vi "Create_Analogue_Time_Array.vi"(0 "Sampling Rate (Hz)":dbl, 1 "Sync Delay (s)":dbl, 2 "No of Samples":i32, 3 "Index":i32, 4 "Total No of Chs":i32) -> (5 "Times":dbl[](array[numeric]))   [LabVIEW 2017]
uses:
  Globals/Meas_global.vi
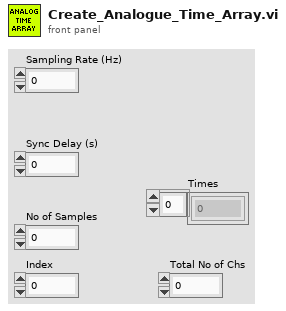
[diagram p1: front panel]
types:
  T1 = typedef "Trigger_Mode.ctl" = enum16{"Free Running", "Start on Trigger", "Trigger Every Block", "Trigger Every Sample"}
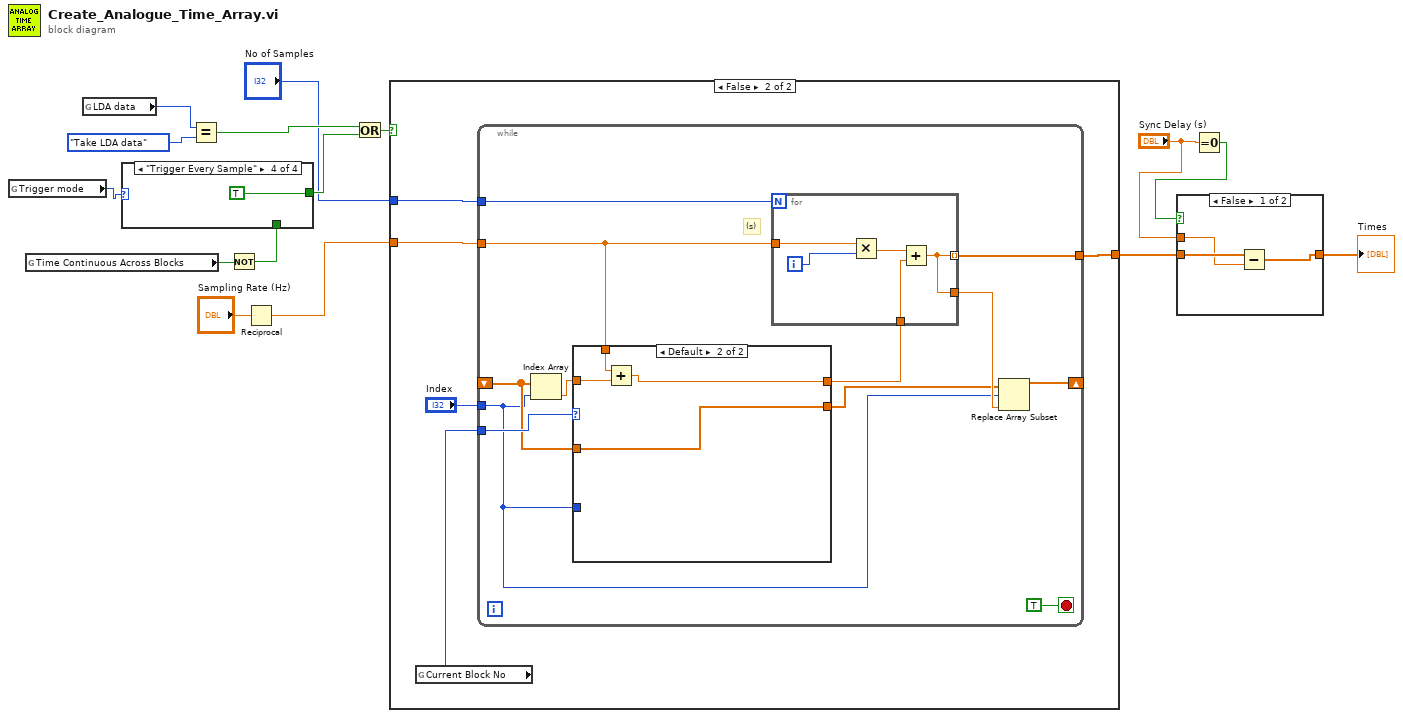
[diagram p0: block diagram]
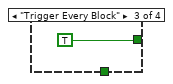
[diagram p5: hidden frame]
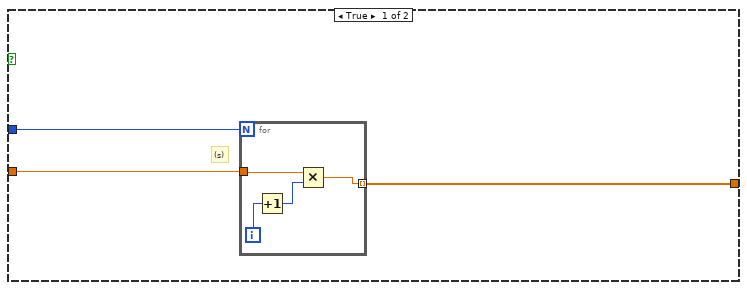
[diagram p6: hidden frame]
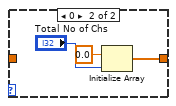
[diagram p8: hidden frame]
diagram:
  n1 = global read "Meas_global.vi" "Trigger mode"() -> (w14:T1)
  n2 = global read "Meas_global.vi" "Time Continuous Across Blocks"() -> (w9:bool)
  n3 = global read "Meas_global.vi" "LDA data"() -> (w6:enum16{"No LDA data", "Take LDA data"})
  n4 = Equal?(x=w6, y=enum16{"No LDA data", "Take LDA data"}."Take LDA data" ("LDA data")) -> (x = y?=w11:bool)
  n5 = Not(x=w9) -> (.not. x?=w8:bool)
  n6 = case shown="\"Trigger Every Sample\"" w14 {
    tunnel: [w16 w17 TRUE TRUE] -> w10
    tunnel: w8 -> [w16 w17 _ _]
    frame "Free Running" {
    }
    frame "Start on Trigger" {
    }
    frame "Trigger Every Block" {
    }
    frame "Trigger Every Sample" {
    }
  }
  n7 = Reciprocal(x="Sampling Rate (Hz)") -> (1/x=w15:dbl)
  n8 = Or(x=w11, y=w10) -> (x .or. y?=w12:bool)
  n9 = case shown="False" w12 {
    tunnel: [w22 w31] -> w2
    tunnel: "No of Samples" -> [w21 w30]
    tunnel: w15 -> [w20 w29]
    frame True {
      # "(s)"
      n10 = for {
        N: w21 -> [_]
        tunnel: w20 -> [w25]
        tunnel: [w24] -> w22 mode=indexing
        i -> [w26]
        n11 = Increment(x=w26) -> (x+1=w23:i32)
        n12 = Multiply(x=w25, y=w23) -> (x*y=w24:dbl)
      }
    }
    frame False {
      n13 = global read "Meas_global.vi" "Current Block No"() -> (w28:i32)
      n14 = while {
        tunnel: [w43] -> w31
        tunnel: w30 -> [w39]
        tunnel: w29 -> [w41]
        shift-right: [w38] -> _
        shift-left: _ -> [w33]
        tunnel: w28 -> [w40]
        tunnel: "Index" -> [w32]
        stop <- TRUE stop-if-true
        # "(s)"
        n15 = Index Array(array=w33, index=w32) -> (element=w36:dbl)
        n16 = case shown="Default" w40 {
          tunnel: [w47 w53] -> w37
          tunnel: w36 -> [_ w55]
          tunnel: w41 -> [w47 w54]
          tunnel: [w46 w52] -> w34
          tunnel: w33 -> [w44 w52]
          tunnel: w32 -> [w45 _]
          frame 1 {
            n17 = case shown="Default" w45 {
              tunnel: [w48 w49] -> w46
              tunnel: w44 -> [w48 _]
              frame Default {
              }
              frame 0 {
                n18 = Initialize Array(0.0 ("element"), "Total No of Chs") -> (w49:dbl[])
              }
            }
          }
          frame Default {
            n19 = Add(x=w54, y=w55) -> (x+y=w53:dbl)
          }
        }
        n20 = for {
          N: w39 -> [_]
          tunnel: w41 -> [w60]
          tunnel: [w57] -> w43 mode=indexing
          tunnel: w37 -> [w58]
          tunnel: [w57] -> w35
          i -> [w56]
          n21 = Multiply(x=w60, y=w56) -> (x*y=w59:dbl)
          n22 = Add(x=w59, y=w58) -> (x+y=w57:dbl)
        }
        n23 = Replace Array Subset(array=w34, new element=w35, index=w32) -> (w38:dbl[])
      }
    }
  }
  n24 = Equal To 0?(x="Sync Delay (s)") -> (x = 0?=w4:bool)
  n25 = case shown="False" w4 {
    tunnel: [w62 w64] -> w3
    tunnel: w2 -> [w63 w64]
    tunnel: "Sync Delay (s)" -> [w61 _]
    frame False {
      n26 = Subtract(x=w63, y=w61) -> (x-y=w62:dbl[])
    }
    frame True {
    }
  }
  "Times" <- w3
